vi "Calibration.vi"(6 "Enable":bool, 7 "New value":sgl format="%#_13g", 8 "error in":errorcluster, 9 "Mode":enum16{"Temperature", "Pressure"}(ring), 10 "Cluster":T1, 11 "VISA Refnum in":refnum<visa-resource-name>) -> (0 "error out":errorcluster, 2 "Cluster Out":T1, 3 "VISA out":refnum<visa-resource-name>)   [LabVIEW 2020]
uses:
  07d31b0d-cea6-448d-a82c-83bef5cfe5dc.vi
  bd00d1ba-4a42-4b12-b8dd-01a27f596110.vi
  <vilib>/NI Modbus.llb/MB Serial Master Query (poly).vi
  MB Serial Master Query Write Single Register (poly).vi
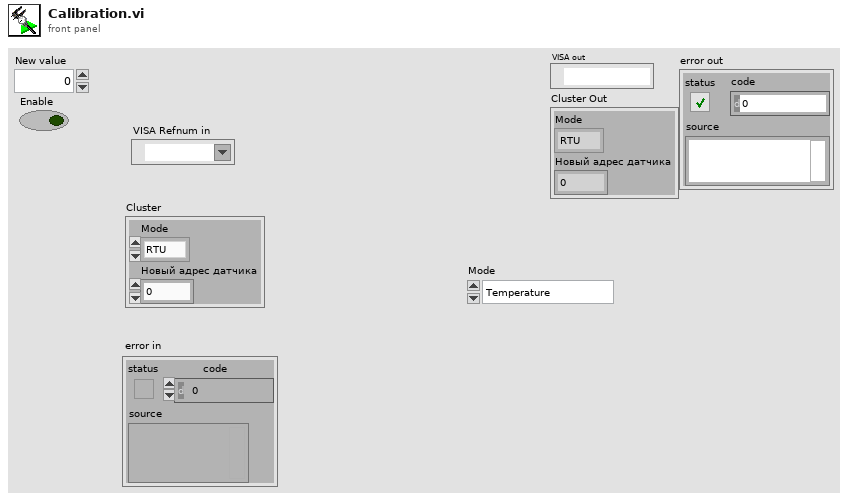
[diagram p1: front panel]
types:
  T1 = cluster{"Mode":enum16{"RTU", "ASCII"}, "Новый адрес датчика":u16}
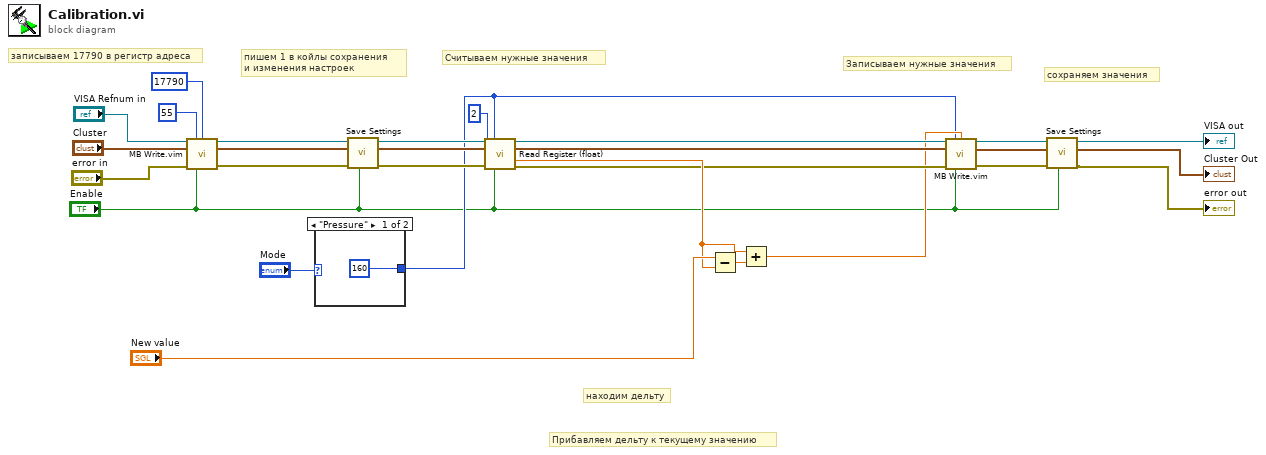
[diagram p0: block diagram]
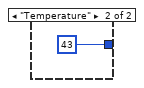
[diagram p2: hidden frame]
diagram:
  # "сохраняем значения"
  # "Записываем нужные значения"
  # "Прибавляем дельту к текущему значению"
  # "находим дельту"
  # "Считываем нужные значения"
  # "пишем 1 в койлы сохранения \nи изменения настроек"
  # "записываем 17790 в регистр адреса"
  n1 = call "MB Write.vim"("VISA Refnum in"="VISA Refnum in", "Command"=u16 55, "Data"=u16 17790, "Cluster"="Cluster", "error in"="error in", "Enable"="Enable") -> ("VISA out"=w19:refnum<visa-resource-name>, "Cluster Out"=w17:T1, "error out"=w15:errorcluster)  [unwired: 7 in]
  n2 = case shown="\"Pressure\"" "Mode" {
    tunnel: [u16 160 ("startReg") u16 43 ("startReg")] -> w8
    frame "Pressure" {
    }
    frame "Temperature" {
    }
  }
  n3 = call "Save Settings.vi"("Enable"="Enable", "error in"=w15, "Cluster"=w17, "VISA Refnum in"=w19) -> ("error out"=w14:errorcluster, "Cluster Out"=w16:T1, "VISA out"=w18:refnum<visa-resource-name>)  [unwired: 5 in]
  n4 = call "Read Register (float).vi"("Refnum in"=w18, "startReg"=w8, "Mode"=w16, "WordCount"=u16 2 ("Quantity"), "error in (no error)"=w14, "Enable"="Enable") -> ("Refnum Out"=w12:refnum<visa-resource-name>, "ModeOut"=w11:T1, "first element"=w13:sgl, "error out"=w10:errorcluster)  [unwired: 5 in, 1 out]
  n5 = Subtract(x="New value", y=w13) -> (x-y=w20:sgl)
  n6 = Add(x=w13, y=w20) -> (x+y=w9:sgl)
  n7 = call "MB Write.vim"("VISA Refnum in"=w12, "Command"=w8, "Data"=w9, "Cluster"=w11, "error in"=w10, "Enable"="Enable") -> ("VISA out"=w7:refnum<visa-resource-name>, "Cluster Out"=w5:T1, "error out"=w4:errorcluster)  [unwired: 7 in]
  n8 = call "Save Settings.vi"("Enable"="Enable", "error in"=w4, "Cluster"=w5, "VISA Refnum in"=w7) -> ("error out"=→"error out":errorcluster, "Cluster Out"=→"Cluster Out":T1, "VISA out"=→"VISA out":refnum<visa-resource-name>)  [unwired: 5 in]
